vi "get enumerate device serial.vi"(8 "error in (no error)":errorcluster, 9 "serial":u32, 10 "device_index":i32, 11 "device_enumeration":u32) -> (0 "error out":errorcluster, 1 "serial out":u32, 3 "function return":i32)   [LabVIEW 2012, in "libximc.lvlib"]
doc: "result_t XIMC_API get_enumerate_device_serial(device_enumeration_t device_enumeration, int device_index, uint32_t* serial);"
uses:
  libximc.lvlib
  libximc.dll
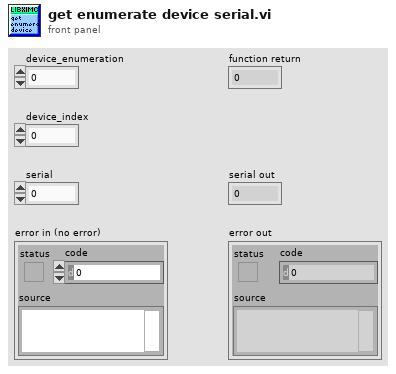
[diagram p1: front panel]
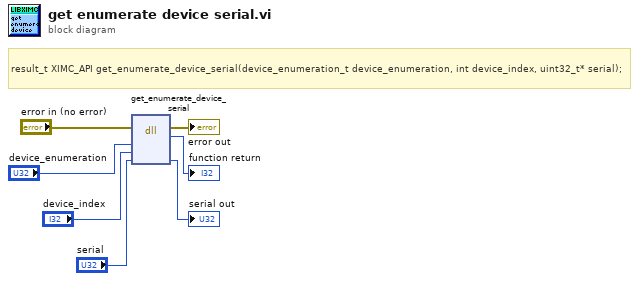
[diagram p0: block diagram]
diagram:
  # "result_t XIMC_API get_enumerate_device_serial(device_enumeration_t device_enumeration, int device_index, uint32_t* serial);"
  n1 = dll-call lib="E:/labview-2.12.1-Labview_12.0/ximcLVx32/libximc.*" fn="get_enumerate_device_serial"(error in="error in (no error)", "device_enumeration"="device_enumeration", "device_index"="device_index", "serial"="serial") -> (error out=→"error out":errorcluster, →"function return":i32, "serial"=→"serial out":u32)  [unwired: 4 in, 1 out]
